vi "Tree Get Active Tree.vi"(8 "error in (no error)":errorcluster, 11 "Tree DVR in":refnum<data-value>) -> (0 "error out":errorcluster, 2 "Returned tree out":refnum<data-value>, 3 "Tree DVR out":refnum<data-value>)   [LabVIEW 2012, in "MDSplus.lvlib"]
doc: "Returns the currently opened and active tree."
uses:
  <vilib>/MDSplus/Library/MDSplus.lvlib
  <vilib>/MDSplus/Classes/Tree_Class/Tree.lvclass
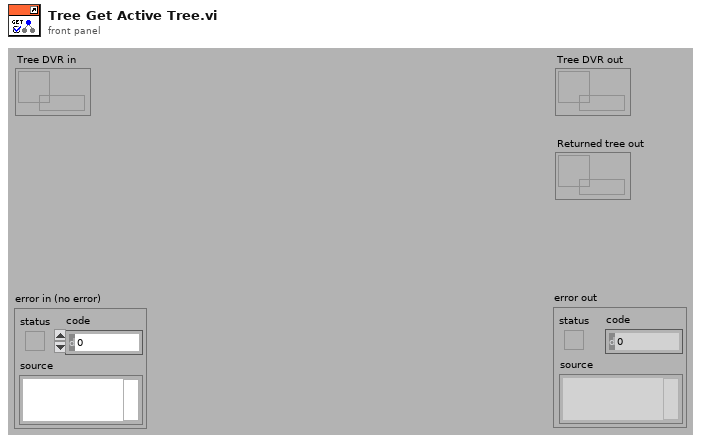
[diagram p1: front panel]
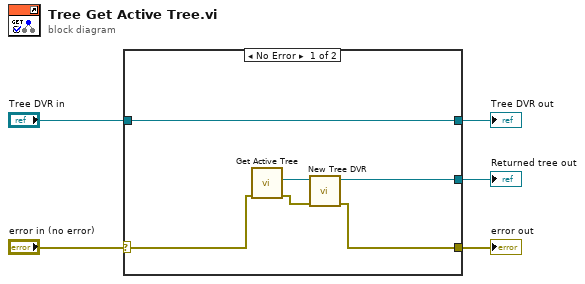
[diagram p0: block diagram]
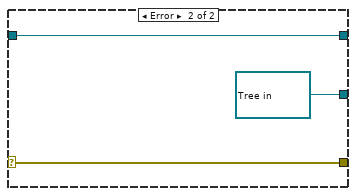
[diagram p2: hidden frame]
diagram:
  n1 = case shown="No Error" "error in (no error)" {
    selector: "error in (no error)" -> [w10 w14]
    tunnel: "Tree DVR in" -> [w11 w13]
    tunnel: [w6 w14] -> w5
    tunnel: [w11 w13] -> w2
    tunnel: [w7 refnum<data-value> refnum ("Tree DVR out")] -> w1
    frame No Error {
      n2 = call <vilib>:"Get Active Tree.vi"("error in (no error)"=w10) -> ("error out"=w8:errorcluster, "Returned tree out"=w9:refnum<class "Tree.lvclass">)  [unwired: 8 in, 1 out]
      n3 = call <vilib>:"New Tree DVR.vi"("error in (no error)"=w8, "Tree in"=w9) -> ("error out"=w6:errorcluster, "Tree DVR out"=w7:refnum<data-value>)  [unwired: 8 in]
    }
    frame Error {
    }
  }
  "error out" <- w5
  "Tree DVR out" <- w2
  "Returned tree out" <- w1
